vi "Lvi Set Triggered Scan.vi"(5 "RetriggerFrequency":dbl, 6 "RetriggerSource":i32, 7 "MultiscanCount":u32, 8 "error in (no error)":errorcluster, 9 "RetriggerMode":i32, 10 "UseTrigScan":bool=TRUE, 11 "TaskRef":i32) -> (0 "error out":errorcluster, 2 "function return":i32, 3 "TaskRef out":i32)   [LabVIEW 2022 SP3, in "DtLvLink.lvlib"]
doc: "Calls directly into the entry points of the DLL of the Data Acq SDK to specify a triggered scan operation for an analog input task. This VI is used by the higher-level VI, DtOLTrigger."
uses:
  DtLvLink.lvlib
  <userlib>/LV-Link3/DtLvLink_64.dll
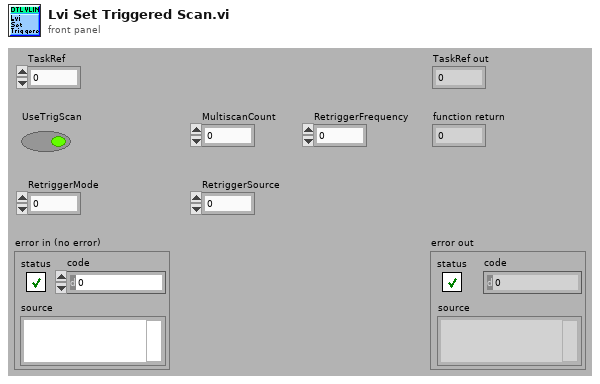
[diagram p1: front panel]
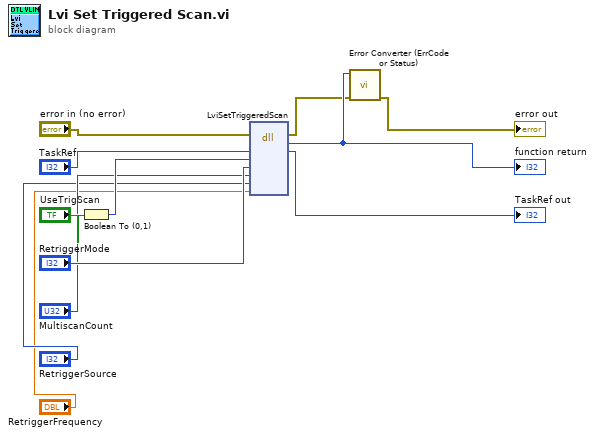
[diagram p0: block diagram]
diagram:
  n1 = Boolean To (0,1)(Boolean="UseTrigScan") -> (0, 1=w8:i16)
  n2 = dll-call lib="C:/Program Files/National Instruments/LabVIEW 2022/user.lib/LV-Link3/DtLvLink_64.*" fn="LviSetTriggeredScan"(error in="error in (no error)", "TaskRef"="TaskRef", "UseTrigScan"=w8, "RetriggerMode"="RetriggerMode", "MultiscanCount"="MultiscanCount", "RetriggerSource"="RetriggerSource", "RetriggerFrequency"="RetriggerFrequency") -> (error out=w2:errorcluster, "return type"=w12:i32, "TaskRef"=→"TaskRef out":i32)  [unwired: 7 in, 1 out]
  "function return" <- w12
  n3 = call "Error Converter (ErrCode or Status).vi"("error in (no error)"=w2, "error code"=w12) -> ("error out"=→"error out":errorcluster)  [unwired: 9 in]
